vi "CHRES Summer 2025 Waveform Generation.vi"() -> ()   [LabVIEW 2020]
uses:
  <vilib>/measure/NI_MABase.lvlib
panel:
  out "Waveform Graph 5":dynamicdata(graph)
  out "t0 2":timestamp
  out "dt":dbl
  out "t0":timestamp
  out "Waveform Graph 4":waveform(dbl)(graph)
  out "output waveform":waveform(dbl)
  out "Array 3":dbl[](array[numeric])
  out "size(s)":i32
  out "Array 2":dynamicdata[](array[waveform])
  out "Array":dynamicdata[](array[waveform])
  out "Waveform Graph 3":dynamicdata(graph)
  in  "stop":bool
  out "signal out":waveform(dbl)
  in  "Slide":dbl(slide) scale=0.0..10000.0
  out "Waveform Graph":waveform(dbl)[](graph)
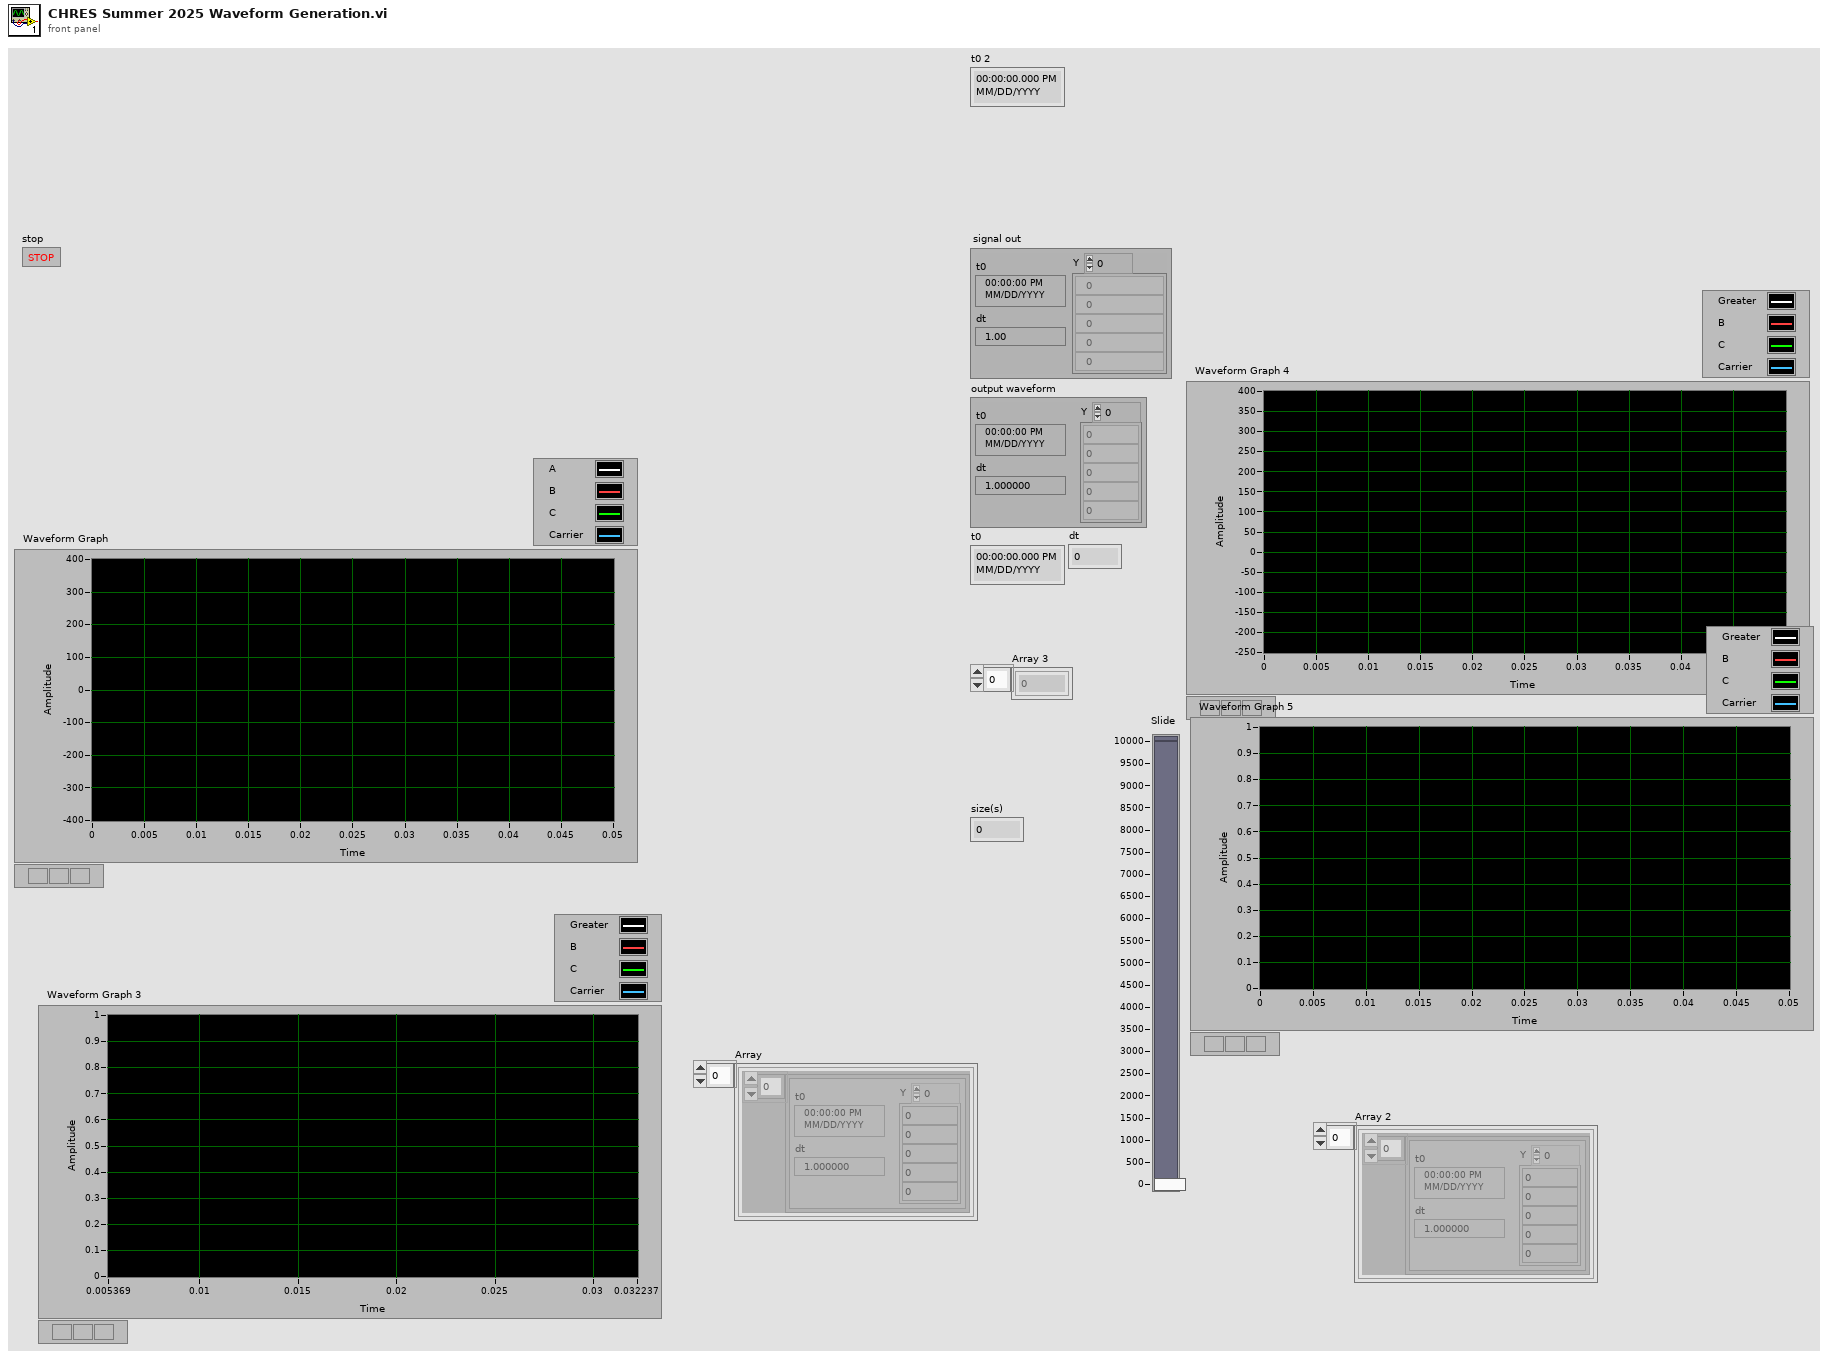
[diagram p1: front panel]
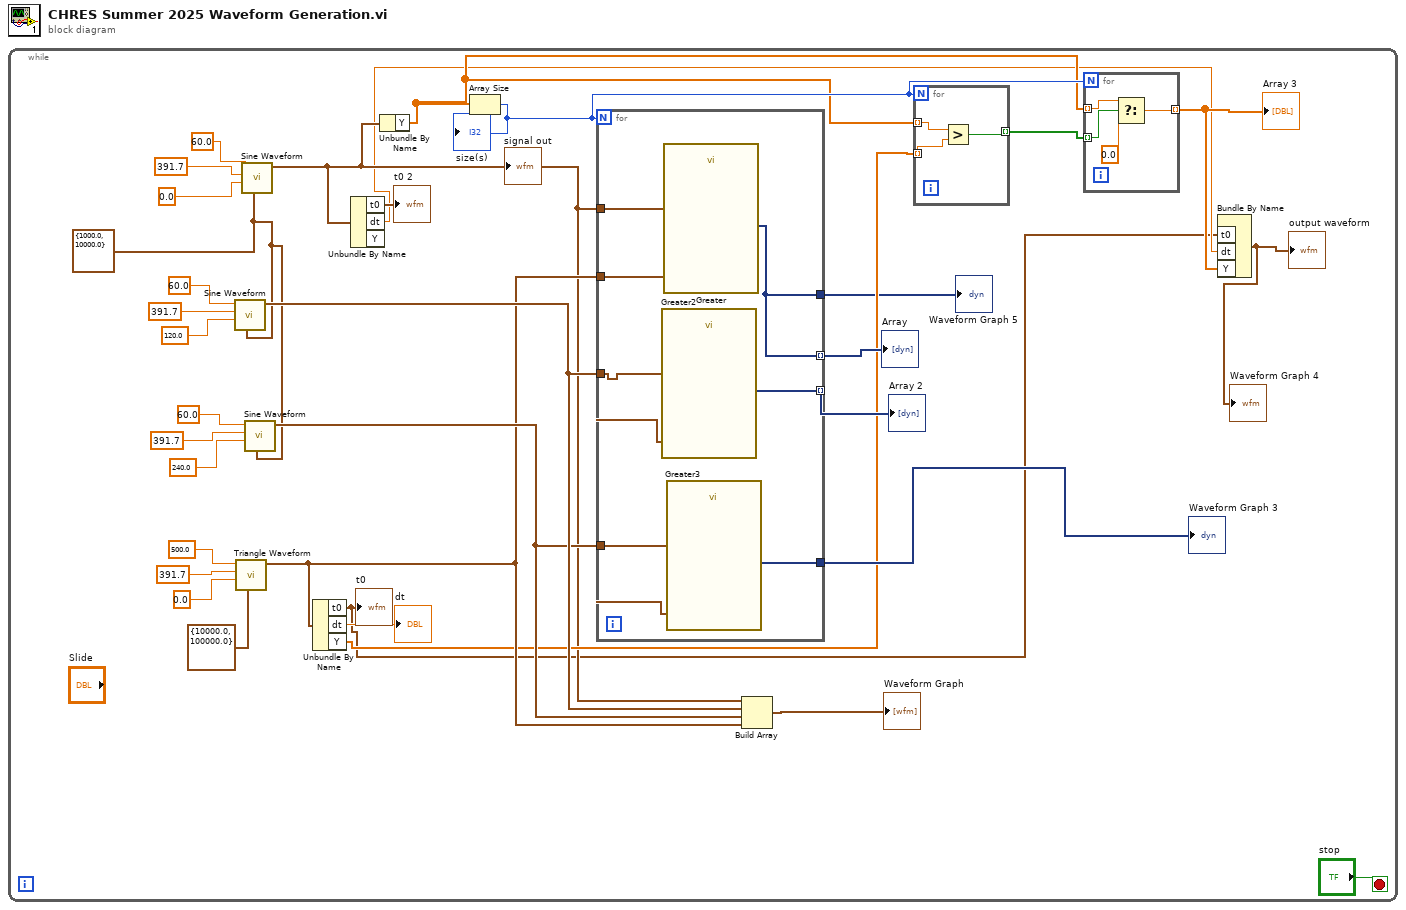
[diagram p0: block diagram]
diagram:
  n1 = while {
    stop <- "stop" stop-if-true
    w18 = cluster{"Fs":dbl, "#s":dbl} {"Fs"=1000.0, "#s"=10000.0} ("sampling info")
    n2 = call <vilib>:"Sine Waveform.vi"("sampling info"=w18, "phase"=120.0, "amplitude"=391.7, "frequency"=60.0) -> ("signal out"=w24:waveform(dbl))  [unwired: 6 in, 1 out]
    n3 = call <vilib>:"Triangle Waveform.vi"("sampling info"=cluster{"Fs":dbl, "#s":dbl} {"Fs"=10000.0, "#s"=100000.0}, "phase"=0.0, "amplitude"=391.7, "frequency"=500.0) -> ("signal out"=w13:waveform(dbl))  [unwired: 6 in, 1 out]
    n4 = call <vilib>:"Sine Waveform.vi"("sampling info"=w18, "phase"=0.0, "amplitude"=391.7, "frequency"=60.0) -> ("signal out"=w6:waveform(dbl))  [unwired: 6 in, 1 out]
    "signal out" <- w6
    n5 = call <vilib>:"Sine Waveform.vi"("sampling info"=w18, "phase"=240.0, "amplitude"=391.7, "frequency"=60.0) -> ("signal out"=w23:waveform(dbl))  [unwired: 6 in, 1 out]
    n6 = Unbundle By Name(w13) -> ("t0"=w2:timestamp, "dt"=→"dt":dbl, "Y"=w12:dbl[])
    "t0" <- w2
    n7 = Unbundle By Name(w6) -> ("t0"=→"t0 2":timestamp, "dt"=w4:dbl)  [unwired: 1 out]
    n8 = Unbundle By Name(w6) -> ("Y"=w9:dbl[])
    n9 = Array Size(array=w9) -> (size(s)=w10:i32)
    "size(s)" <- w10
    n10 = for {
      N: w10 -> [_]
      tunnel: w24 -> [w43]
      tunnel: w13 -> [w48]
      tunnel: w23 -> [w47]
      tunnel: w6 -> [w46]
      tunnel: [w45] -> w14 mode=indexing
      tunnel: [w44] -> w16
      tunnel: [w42] -> w15 mode=indexing
      tunnel: [w42] -> w1
      n11 = call "Greater2"("Operand 2"=w48, "Operand 1"=w43) -> ("Result"=w45:dynamicdata)  [unwired: 8 in, 1 out]
      n12 = call "Greater"("Operand 2"=w48, "Operand 1"=w46) -> ("Result"=w42:dynamicdata)  [unwired: 8 in, 1 out]
      n13 = call "Greater3"("Operand 2"=w48, "Operand 1"=w47) -> ("Result"=w44:dynamicdata)  [unwired: 8 in, 1 out]
    }
    "Waveform Graph 3" <- w16
    "Array" <- w15
    "Array 2" <- w14
    "Waveform Graph 5" <- w1
    n14 = Build Array(w6, w24, w23, w13) -> (→"Waveform Graph":waveform(dbl)[])
    n15 = for {
      N: w10 -> [_]
      tunnel: w9 -> [w41] mode=indexing
      tunnel: w12 -> [w40] mode=indexing
      tunnel: [w39] -> w11 mode=indexing
      n16 = Greater?(x=w41, y=w40) -> (0:w39:bool)
    }
    n17 = for {
      N: w10 -> [_]
      tunnel: w11 -> [w38] mode=indexing
      tunnel: w9 -> [w37] mode=indexing
      tunnel: [w35] -> w8 mode=indexing
      n18 = Select(t=w37, s=w38, f=0.0) -> (s? t:f=w35:dbl)
    }
    "Array 3" <- w8
    n19 = Bundle By Name("t0"=w2, "dt"=w4, "Y"=w8) -> (→"output waveform" →"Waveform Graph 4":waveform(dbl))  [unwired: 1 in]
  }
